vi "总磷流程质控自动启动.vi"(10 "总磷量程切换":enum32{"H", "L", "AUTO"}(ring)=enum."AUTO", 11 "参数":T1={"是否启用仪器"=FALSE, "CODMn"={"启动测量模式"={"测量模式"=enum."水样测量"}, "确定按钮"=TRUE}, "启动模块"={"氨氮"=FALSE, "总磷"=FALSE, "总氮"=FALSE, "COD"=FALSE}, "常规启动"=FALSE, "直接启动"=FALSE}) -> ()   [LabVIEW 2016, in "质控单元.lvlib"]
panel:
  out "枚举 2":enum16{"初始化", "采配水启动", "等待", "配水", "排水", "结束"}(ring)
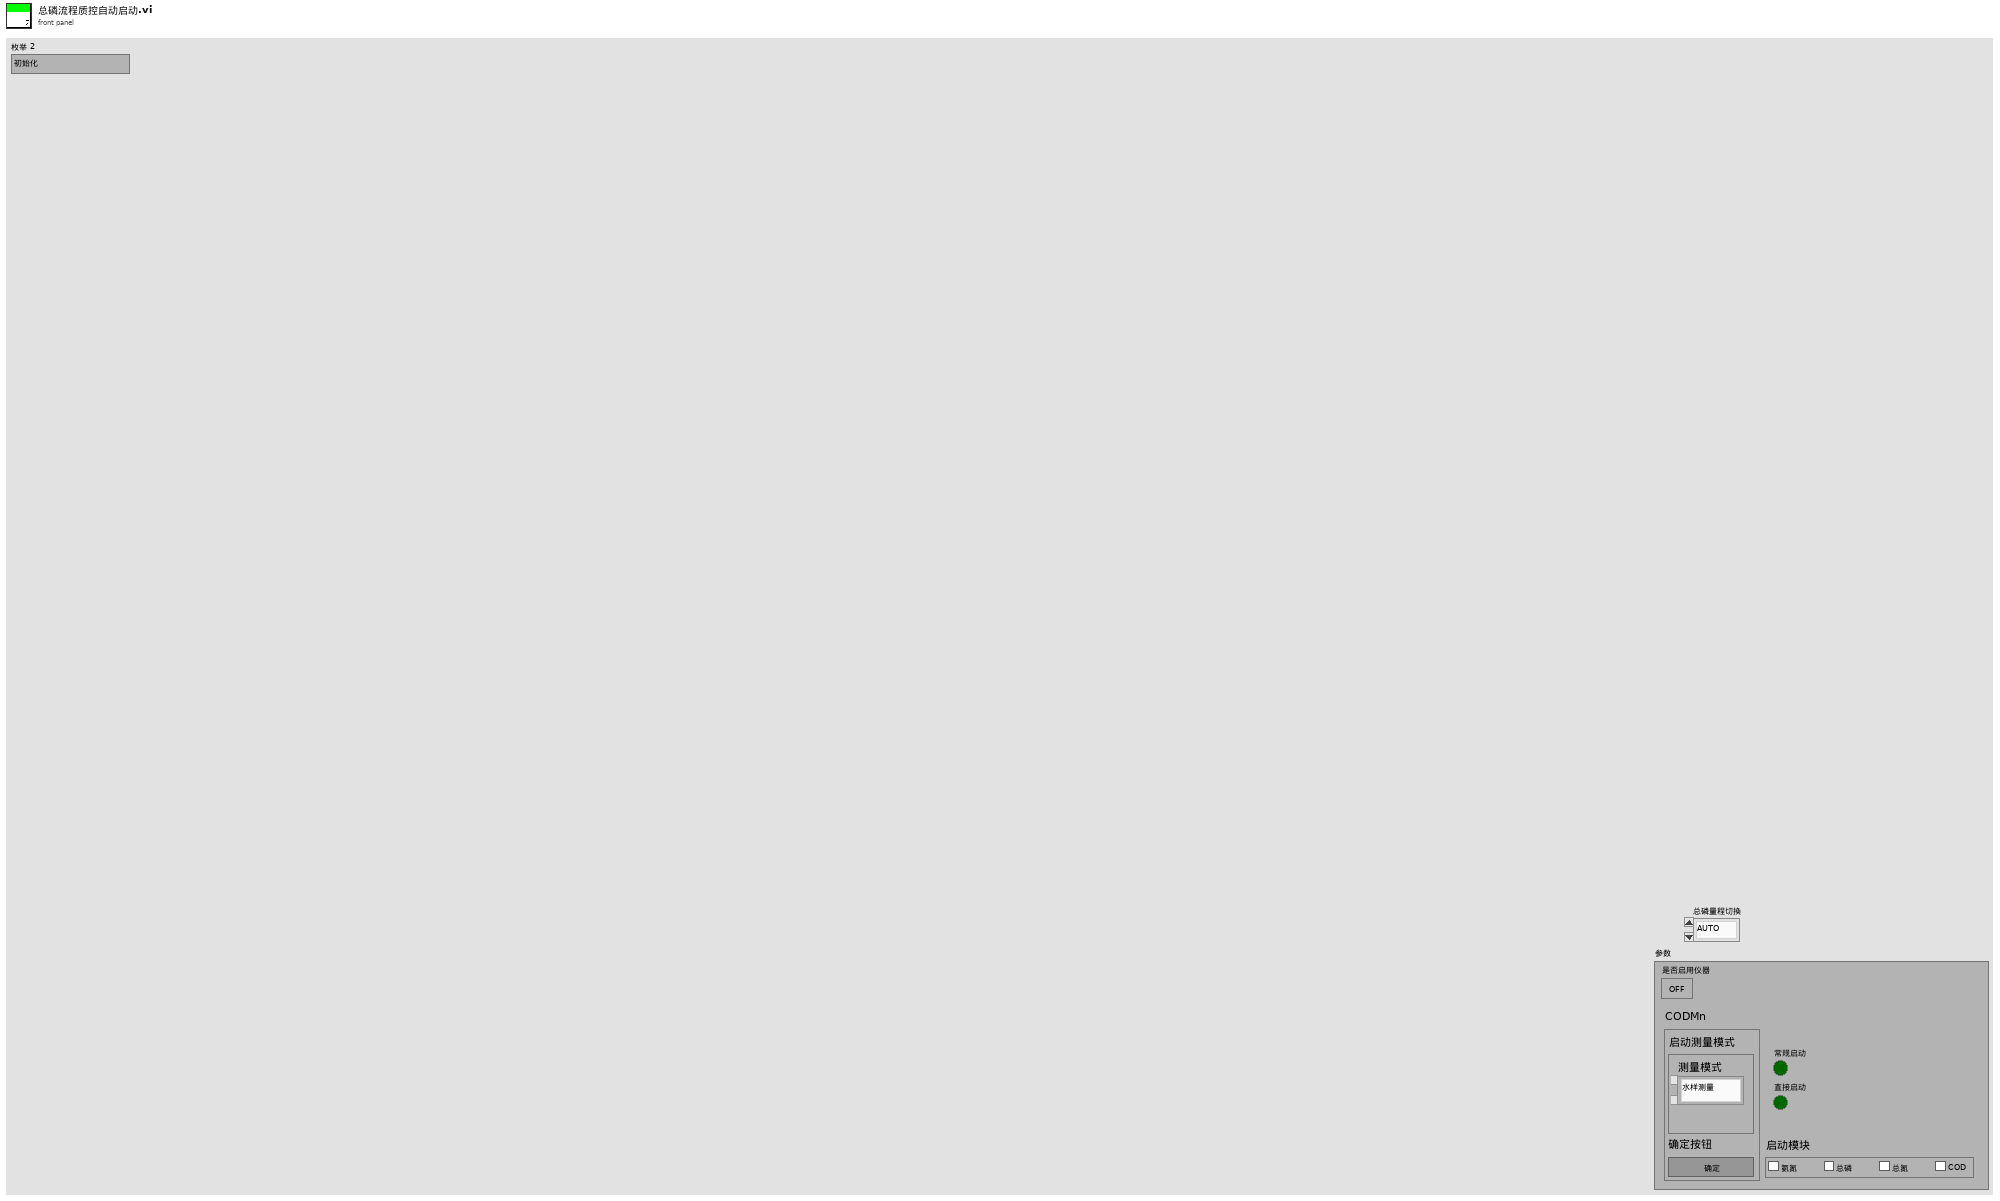
[diagram p1: front panel]
types:
  T1 = cluster{"是否启用仪器":bool, "CODMn":cluster{"启动测量模式":cluster{"测量模式":enum16{"水样测量", "标样核查", "加标回收", "平行样", "校零", "校标"}}, "确定按钮":bool}, "启动模块":cluster{"氨氮":bool, "总磷":bool, "总氮":bool, "COD":bool}, "常规启动":bool, "直接启动":bool}
  T2 = cluster{"R0":i16, "R1":i16, "R2":i16, "R3":i16, "R4":i16, "R5":i16, "R6":i16, "R7":i16, "R8":i16, "R9":i16, "R10":i16, "R11":i16, "R12":i16, "R13":i16, "R14":i16, "R15":i16, "R16":i16, "R17":i16, "R18":i16, "R19":i16, "R20":i16, "R21":i16, "R22":i16, "R23":i16, "R24":i16, "R25":i16, "R26":i16, "R27":i16, "R28":i16, "R29":i16, "R30":i16, "R31":i16, "R32":i16, "R33":i16, "R34":i16, "R35":i16, "R36":i16, "R37":i16, "R38":i16, "R39":i16, "R40":i16, "R41":i16, "R42":i16, "R43":i16, "R44":i16, "R45":i16, "R46":i16, "R47":i16, "R48":i16, "R49":i16, "R50":i16, "R51":i16, "R52":i16, "R53":i16, "R54":i16, "R55":i16, "R56":i16}
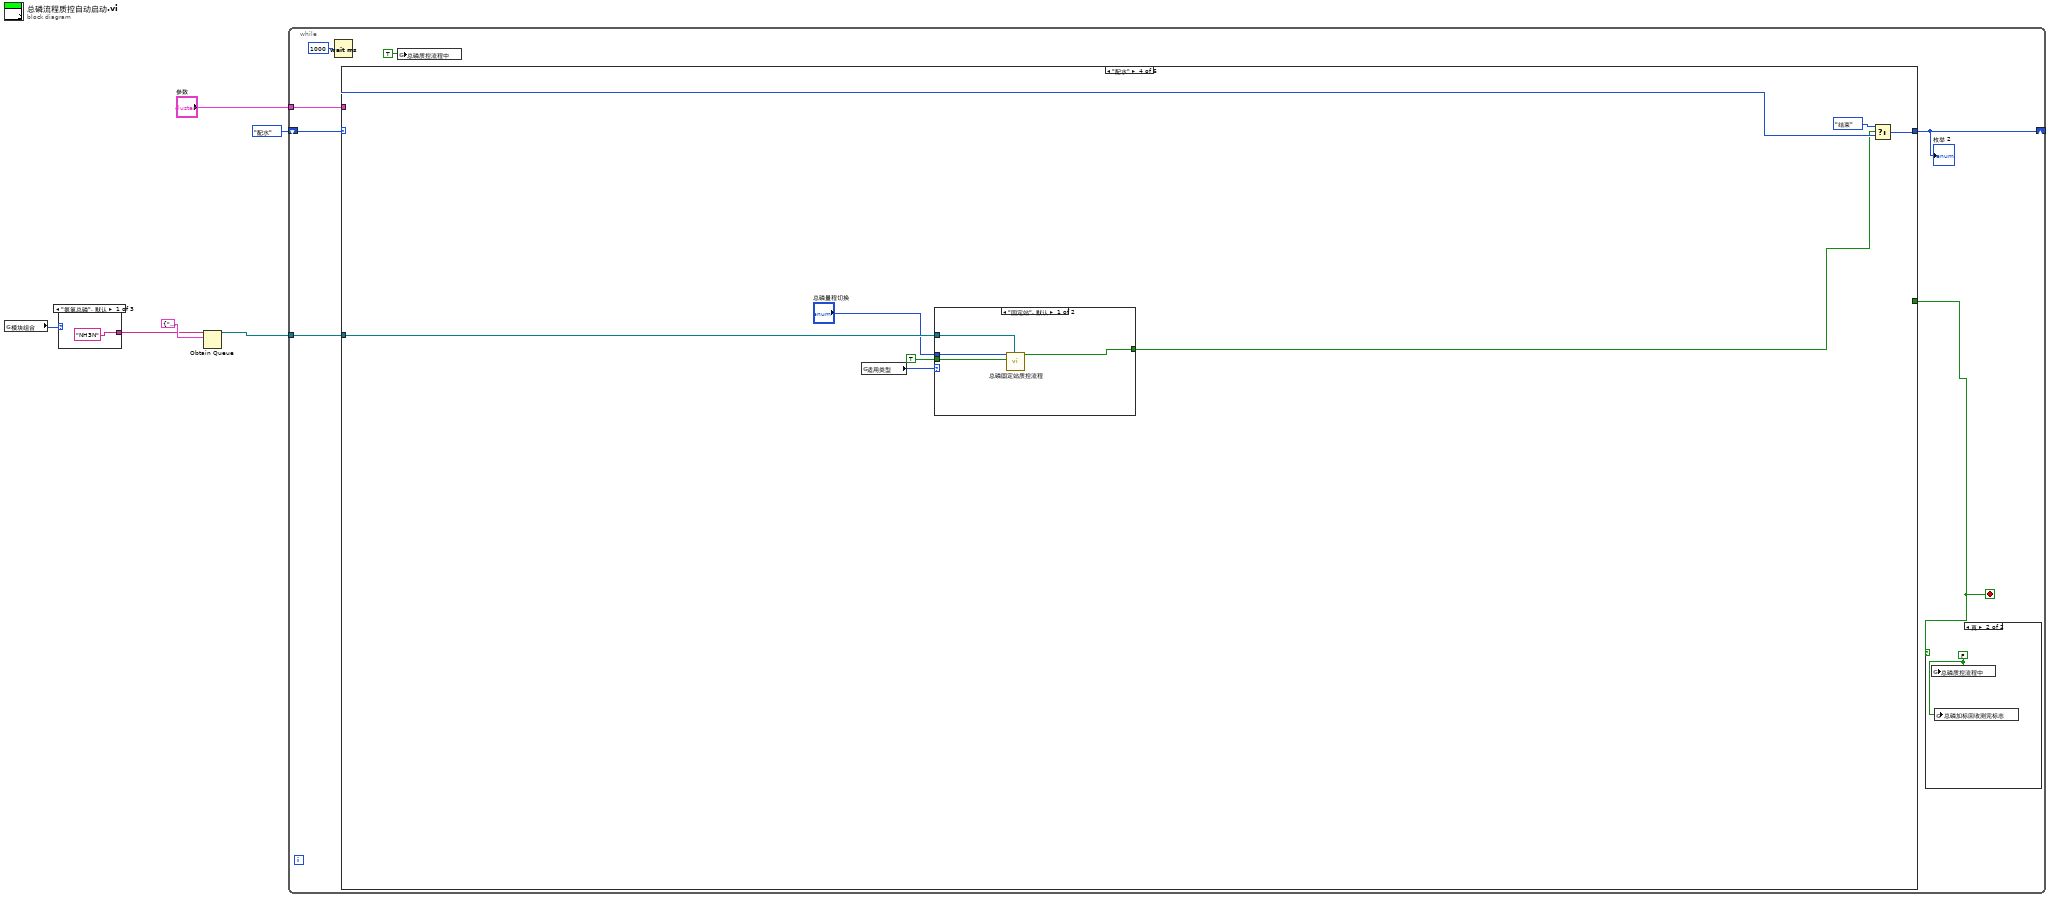
[diagram p0: block diagram]
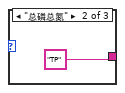
[diagram p2: hidden frame]
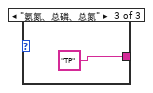
[diagram p3: hidden frame]
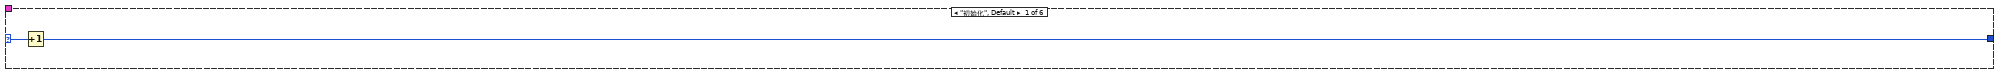
[diagram p5: hidden frame]
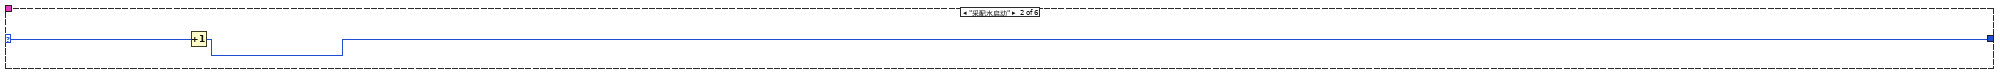
[diagram p6: hidden frame]
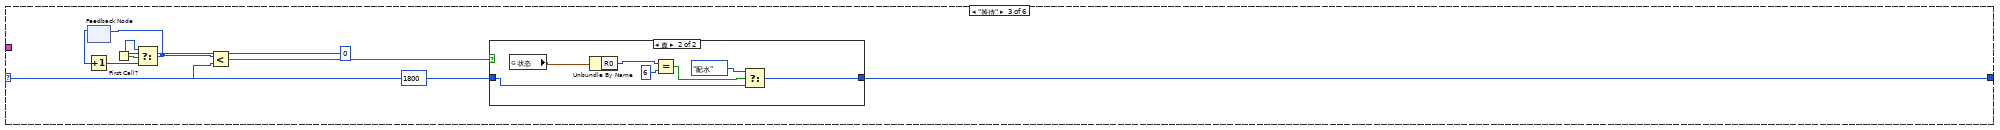
[diagram p7: hidden frame]
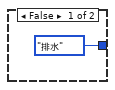
[diagram p8: hidden frame]
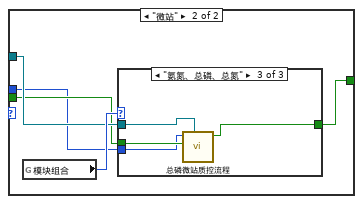
[diagram p9: hidden frame]
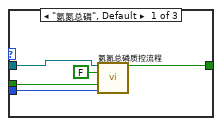
[diagram p10: hidden frame]
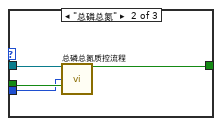
[diagram p11: hidden frame]
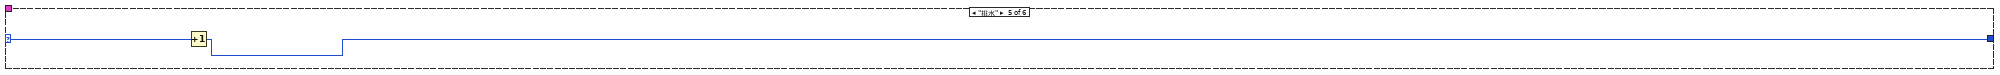
[diagram p12: hidden frame]
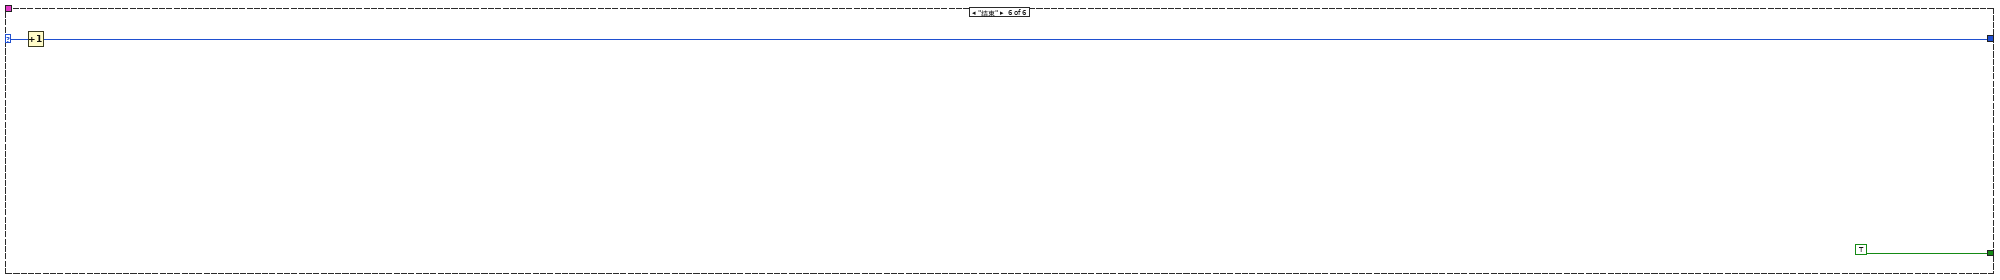
[diagram p13: hidden frame]
diagram:
  n1 = global read "断电保存全局.vi" "模块组合"() -> (w2:enum16{"氨氮总磷", "总磷总氮", "氨氮、总磷、总氮"})
  n2 = case shown="\"氨氮总磷\", 默认" w2 {
    tunnel: ["NH3N" ("名称（未命名）") "TP" ("名称（未命名）") "TP" ("名称（未命名）")] -> w1
    frame "氨氮总磷", Default {
    }
    frame "总磷总氮" {
    }
    frame "氨氮、总磷、总氮" {
    }
  }
  n3 = Obtain Queue(name (unnamed)=w1, element data type=cluster{"命令":string, "data":variant} {"命令"="", "data"=variant}) -> (queue out=w3:refnum<queue>)  [unwired: 3 in, 2 out]
  n4 = while {
    shift-right: [w15] -> _
    shift-left: enum16{"初始化", "采配水启动", "等待", "配水", "排水", "结束"}."配水" ("枚举") -> [w16]
    tunnel: "参数" -> [w13]
    tunnel: w3 -> [w12]
    stop <- w10 stop-if-true
    n5 = Wait (ms)(milliseconds to wait=u32 1000 ("等待时间（毫秒）")) -> ()  [unwired: 1 out]
    n6 = case shown="\"配水\"" w16 {
      selector: w16 -> [w19 w21 w28 w45 w70 w73]
      tunnel: [w18 w20 w27 w44 w69 w72] -> w15
      tunnel: [_ _ _ _ _ TRUE] -> w10
      tunnel: w13 -> [_ _ _ _ _ _]
      tunnel: w12 -> [_ _ _ w43 _ _]
      frame "初始化", Default {
        n7 = Increment(x=w19) -> (x+1=w18:enum16{"初始化", "采配水启动", "等待", "配水", "排水", "结束"})
      }
      frame "采配水启动" {
        n8 = Increment(x=w21) -> (x+1=w20:enum16{"初始化", "采配水启动", "等待", "配水", "排水", "结束"})
      }
      frame "等待" {
        n9 = feedback #1() -> (w24:i32)  [unwired: 1 in]
        n10 = Increment(x=w24) -> (x+1=w23:i32)
        n11 = First Call?() -> (First Call?: T/F=w25:bool)
        n12 = Select(t=0, s=w25, f=w23) -> (s? t:f=w22:i32)
        n13 = feedback-in #1(w22) -> ()
        n14 = Less?(x=w22, y=1800) -> (x < y?=w29:bool)
        n15 = case shown="真" w29 {
          tunnel: w28 -> [_ w34]
          tunnel: [enum16{"初始化", "采配水启动", "等待", "配水", "排水", "结束"}."排水" ("枚举") w33] -> w27
          frame False {
          }
          frame True {
            n16 = global read "与采配水交互全局.vi" "状态"() -> (w32:T2)
            n17 = Unbundle By Name(w32) -> ("R0"=w38:i16)
            n18 = Equal?(x=w38, y=i16 6) -> (x = y?=w36:bool)
            n19 = Select(t=enum16{"初始化", "采配水启动", "等待", "配水", "排水", "结束"}."配水" ("枚举"), s=w36, f=w34) -> (s? t:f=w33:enum16{"初始化", "采配水启动", "等待", "配水", "排水", "结束"})
          }
        }
      }
      frame "配水" {
        n20 = global read "断电保存全局.vi" "适用类型"() -> (w39:enum16{"固定站", "微站"})
        n21 = case shown="\"固定站\", 默认" w39 {
          tunnel: w43 -> [w50 w54]
          tunnel: "总磷量程切换" -> [w49 w52]
          tunnel: TRUE ("氨氮") -> [w48 w53]
          tunnel: [w47 w51] -> w40
          frame "固定站", Default {
            n22 = call "总磷固定站质控流程.vi"("队列输入TP"=w50, "总磷"=w48, "总磷量程切换"=w49) -> ("布尔"=w47:bool)  [unwired: 7 in]
          }
          frame "微站" {
            n23 = global read "断电保存全局.vi" "模块组合"() -> (w55:enum16{"氨氮总磷", "总磷总氮", "氨氮、总磷、总氮"})
            n24 = case shown="\"氨氮、总磷、总氮\"" w55 {
              tunnel: w54 -> [w56 w64 w68]
              tunnel: w53 -> [w60 w62 w67]
              tunnel: w52 -> [w59 w61 w66]
              tunnel: [w57 w63 w65] -> w51
              frame "氨氮总磷", Default {
                n25 = call "氨氮总磷质控流程.vi"("队列输入"=w56, "氨氮"=FALSE, "总磷"=w60, "总磷量程切换"=w59) -> ("布尔"=w57:bool)  [unwired: 9 in, 2 out]
              }
              frame "总磷总氮" {
                n26 = call "总磷总氮质控流程.vi"("队列输入TP"=w64, "总磷量程切换"=w61, "总磷"=w62) -> ("布尔"=w63:bool)  [unwired: 10 in, 2 out]
              }
              frame "氨氮、总磷、总氮" {
                n27 = call "总磷微站质控流程.vi"("队列输入TP"=w68, "总磷"=w67, "总磷量程切换"=w66) -> ("布尔"=w65:bool)  [unwired: 7 in]
              }
            }
          }
        }
        n28 = Select(t=enum16{"初始化", "采配水启动", "等待", "配水", "排水", "结束"}."结束" ("枚举"), s=w40, f=w45) -> (s? t:f=w44:enum16{"初始化", "采配水启动", "等待", "配水", "排水", "结束"})
      }
      frame "排水" {
        n29 = Increment(x=w70) -> (x+1=w69:enum16{"初始化", "采配水启动", "等待", "配水", "排水", "结束"})
      }
      frame "结束" {
        n30 = Increment(x=w73) -> (x+1=w72:enum16{"初始化", "采配水启动", "等待", "配水", "排水", "结束"})
      }
    }
    "枚举 2" <- w15
    n31 = global write "质控测完标志全局 1.vi" "总磷质控流程中"(TRUE ("氨氮质控流程中")) -> ()
    n32 = case shown="真" w10 {
      frame False {
      }
      frame True {
        w17 = FALSE ("氨氮质控流程中")
        n33 = global write "质控测完标志全局 1.vi" "总磷质控流程中"(w17) -> ()
        n34 = global write "质控测完标志全局 1.vi" "总磷加标回收测完标志"(w17) -> ()
      }
    }
  }
